vi "Average Over Period.vi"(2 "Period":dbl[unit], 3 "Cluster":cluster{dbl, dbl, dbl[]}) -> (1 "Average":dbl)   [LabVIEW 2010]
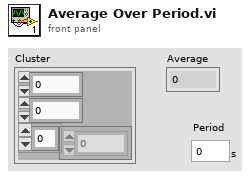
[diagram p1: front panel]
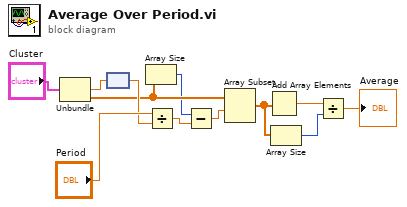
[diagram p0: block diagram]
diagram:
  n1 = Unbundle("Cluster") -> (w11:dbl, w4:dbl[])  [unwired: 1 out]
  n2 = node(w11) -> (w9:dbl[unit])
  n3 = Array Size(array=w4) -> (size(s)=w3:i32)
  n4 = Divide(x="Period", y=w9) -> (x/y=w2:dbl)
  n5 = Subtract(x=w3, y=w2) -> (x-y=w1:dbl)
  n6 = Array Subset(array=w4, index=w1) -> (w8:dbl[])  [unwired: 1 in]
  n7 = Add Array Elements(numeric array=w8) -> (sum=w6:dbl)
  n8 = Array Size(array=w8) -> (size(s)=w5:i32)
  n9 = Divide(x=w6, y=w5) -> (x/y=→"Average":dbl)
